vi "Test Process Unexpected Lifecycle States.vi"(8 "error in (no error)":errorcluster, 11 "Process Test In":refnum<class "Process Test.lvclass">) -> (0 "error out":errorcluster, 3 "Process Test Out":refnum<class "Process Test.lvclass">)   [LabVIEW 2020, in "Process Test.lvclass"]
uses:
  Process Test.lvclass
  C:/Users/anton/Documents/GitHub/Triarc-Framework/source/Framework Test/Base Class Test/Base Test.lvclass
  C:/Program Files (x86)/National Instruments/LabVIEW 2020/vi.lib/Asteme/LUnit/Test Case.lvclass
  Framework/Process/Process.lvclass
  Base Class Test/Base Test.lvclass/Base Test.ctl
  <vilib>/Asteme/LUnit/Test Case.lvclass/Test Case.ctl
  <vilib>/Asteme/LUnit/LUnit Assertion Result.lvclass/LUnit Assertion Result.ctl
  Framework/Process/Process.lvclass/Process.ctl
  <vilib>/Asteme/LUnit/Palette/Fail.vi
  <vilib>/Asteme/LUnit/Palette/Pass.vi
  <vilib>/Asteme/LUnit/Set Assertion Type.vi
  Framework/Process/Public/Lifecycle/Get Lifecycle State.vi
  Framework/Process/Private/SubVIs/Wait for finish.vi
  Framework/Process/Protected/Messaging/Enqueue Message.vi
  Framework/Process/Private/SubVIs/Set Lifecycle State.vi
  <vilib>/Asteme/LUnit/Palette/Pass If.vi
  <vilib>/Asteme/LUnit/Add test result.vi
  <vilib>/Asteme/LUnit/LUnit Write Passed.vi
  <vilib>/Asteme/LUnit/LUnit Get Test Case.vi
  <vilib>/Asteme/LUnit/Assertion Result/LUnit Get Test Name.vi
  <vilib>/Asteme/LUnit/LUnit Write Message.vi
  <vilib>/Asteme/LUnit/LUnit Write Description.vi
  <vilib>/Asteme/LUnit/LUnit Write Assertion Type.vi
  <vilib>/Utility/error.llb/Clear Errors.vi
  <vilib>/Asteme/LUnit/Read Test Case Name.vi
  <vilib>/Utility/error.llb/Error Cluster From Error Code.vi
  Framework/Base/Base.lvclass
  <vilib>/Asteme/LUnit/LUnit Assertion Result.lvclass
  <vilib>/Asteme/LUnit/Test Case.lvclass
  Base Class Test/Base Test.lvclass
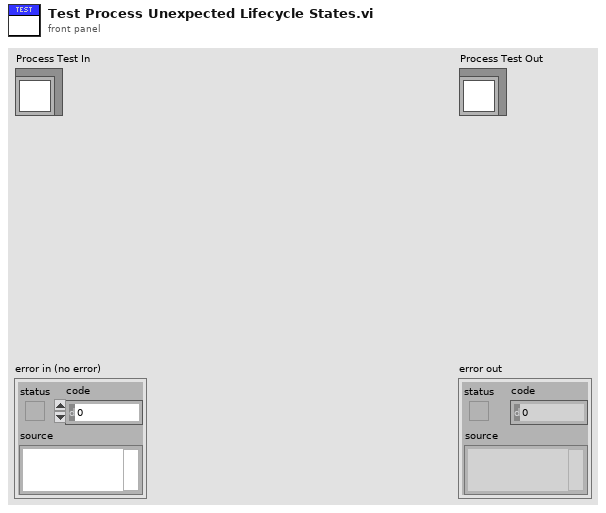
[diagram p1: front panel]
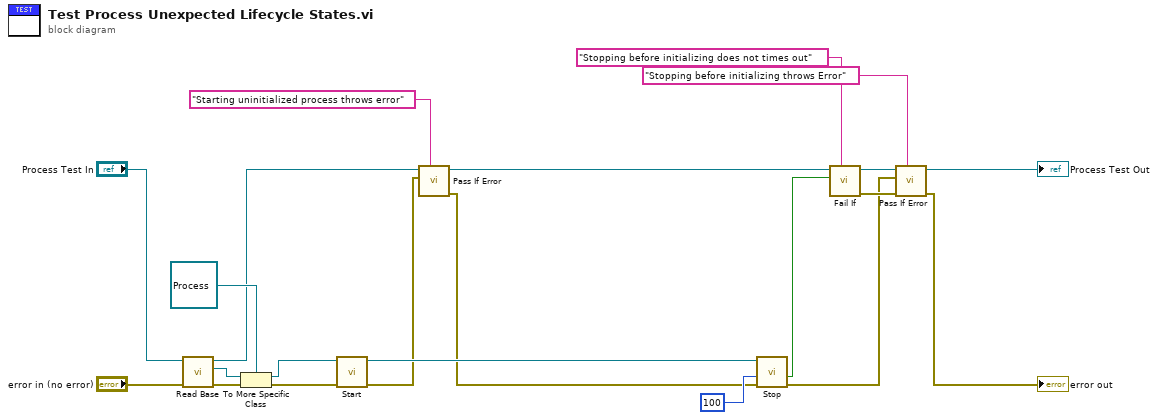
[diagram p0: block diagram]
diagram:
  n1 = call "Read Base.vi"("error in (no error)"="error in (no error)", "Base Class Test In"="Process Test In") -> ("error out"=w8:errorcluster, "Base.lvclass"=w9:refnum<class "Base.lvclass">, "Base Class Test Out"=w4:refnum<class "Process Test.lvclass">)  [unwired: 7 in]
  n2 = To More Specific Class(target class=refnum<class "Process.lvclass"> refnum ("Process.lvclass"), reference=w9, error in=w8) -> (specific class reference=w3:refnum<class "Process.lvclass">, error out=w6:errorcluster)
  n3 = call "Start.vi"("error in (no error)"=w6, "Process In"=w3) -> ("error out"=w18:errorcluster, "Process Out"=w22:refnum<class "Process.lvclass">)  [unwired: 8 in]
  n4 = call <vilib>:"Pass If Error.vi"("Description"="Starting uninitialized process throws error", "Assert error"=w18, "Test Case In"=w4) -> ("error out"=w17:errorcluster, "Test Case Out"=w20:refnum<class "Process Test.lvclass">)  [unwired: 7 in]
  n5 = call "Stop.vi"("error in (no error)"=w17, "timeout in ms (-1)"=100, "Process In"=w22) -> ("error out"=w2:errorcluster, "timed out?"=w16:bool)  [unwired: 6 in, 1 out]
  n6 = call <vilib>:"Fail If.vi"("Description"="Stopping before initializing does not times out", "Fail?"=w16, "Test Case In"=w20) -> ("error out"=w13:errorcluster, "Test Case Out"=w14:refnum<class "Process Test.lvclass">)  [unwired: 7 in]
  n7 = call <vilib>:"Pass If Error.vi"("Description"="Stopping before initializing throws Error", "error in (no error)"=w13, "Assert error"=w2, "Test Case In"=w14) -> ("error out"=→"error out":errorcluster, "Test Case Out"=→"Process Test Out":refnum<class "Process Test.lvclass">)  [unwired: 6 in]
